vi "EISExample.vi"() -> ()   [LabVIEW 2025]
uses:
  PalmSens/PalmSens.lvclass
  PalmSens/MeasurementResults.ctl
  PalmSens/LiveCurveResult.ctl
  E:/PSCode/PalmSens_SDK/labview/PalmSens/Libraries/PalmSens.Core.Simplified.LabVIEW.dll
  PalmSens/Libraries/PalmSens.Core.Simplified.LabVIEW.dll
panel:
  out "Method Indicator":refnum<k24>
  out "Results":T1
  out "Array":string[](array[string])
  out "Is Measuring":bool
  in  "PalmSens.lvclass":refnum<class "PalmSens.lvclass">
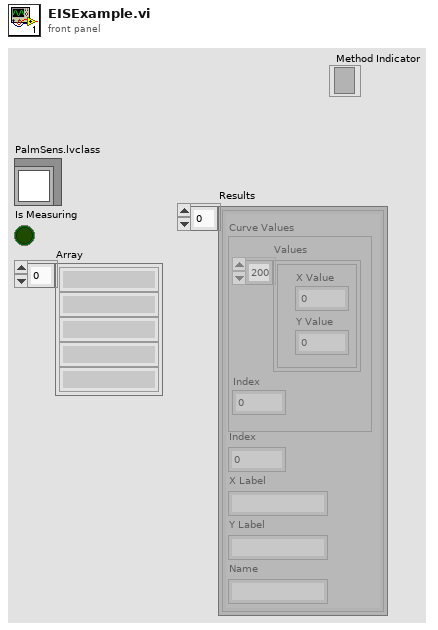
[diagram p1: front panel]
types:
  T1 = typedef "MeasurementResults.ctl" = T2[]
  T2 = typedef "LiveCurveResult.ctl" = cluster{"X Label":string, "Y Label":string, "Name":string, "Index":i16, "Curve Values":cluster{"Values":cluster{"X Value":dbl, "Y Value":dbl}[], "Index":i16}}
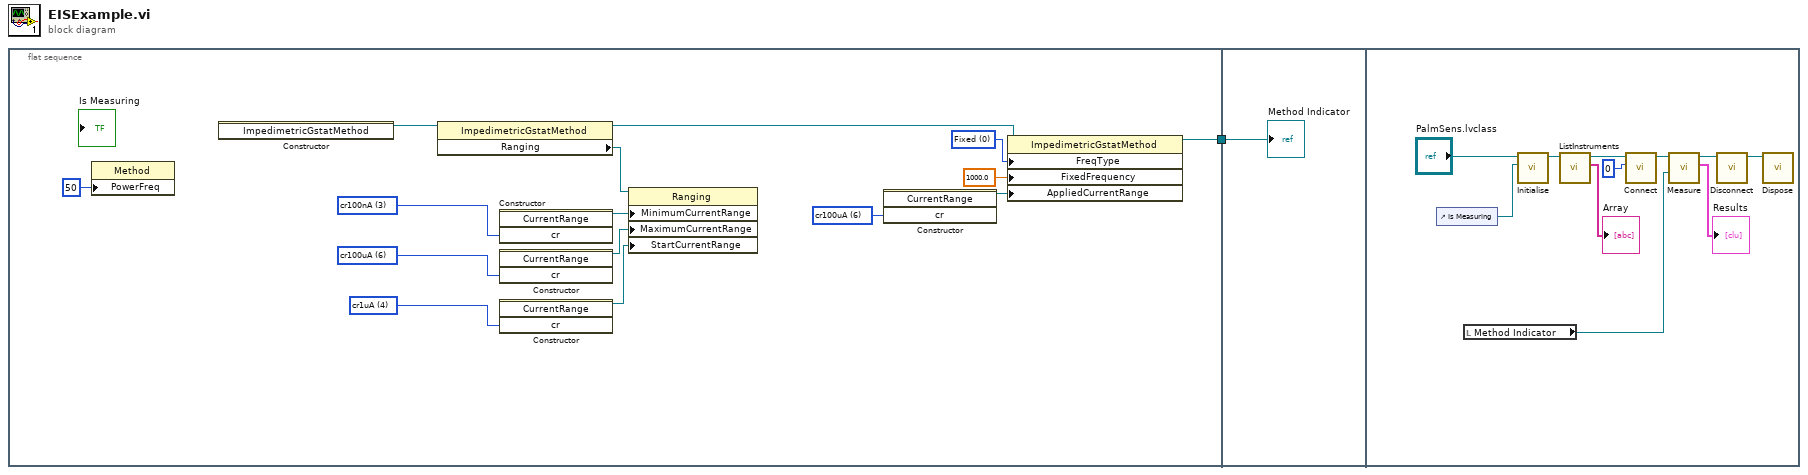
[diagram p0: block diagram]
diagram:
  n1 = flat-sequence {
    tunnel: [w2] -> w1
    tunnel: w1 -> [w17]
    frame #0 {
      w8 = 6 items=["cr100pA"=0, "cr1nA"=1, "cr10nA"=2, "cr100nA"=3, "cr1uA"=4, "cr10uA"=5, "cr100uA"=6, "cr1mA"=7, "cr10mA"=8, "cr100mA"=9, "cr2uA"=10, "cr4uA"=11, "cr8uA"=12, "cr16uA"=13, "cr32uA"=14, "cr125uA"=17, "cr250uA"=18, "cr500uA"=19, "cr5mA"=20, "cr6uA"=21, "cr13uA"=22, "cr25uA"=23, "cr50uA"=24, "cr200uA"=25, "cr63uA"=26, "cr1mA_shunt"=27, "cr10mA_shunt"=28, "cr100mA_shunt"=29, "cr1A"=30, "cr2500uA"=31] ("cr")
      w7 = 0 items=["Fixed", "Scan"] ("FreqType")
      w5 = 4 items=["cr100pA"=0, "cr1nA"=1, "cr10nA"=2, "cr100nA"=3, "cr1uA"=4, "cr10uA"=5, "cr100uA"=6, "cr1mA"=7, "cr10mA"=8, "cr100mA"=9, "cr2uA"=10, "cr4uA"=11, "cr8uA"=12, "cr16uA"=13, "cr32uA"=14, "cr125uA"=17, "cr250uA"=18, "cr500uA"=19, "cr5mA"=20, "cr6uA"=21, "cr13uA"=22, "cr25uA"=23, "cr50uA"=24, "cr200uA"=25, "cr63uA"=26] ("cr")
      w4 = 6 items=["cr100pA"=0, "cr1nA"=1, "cr10nA"=2, "cr100nA"=3, "cr1uA"=4, "cr10uA"=5, "cr100uA"=6, "cr1mA"=7, "cr10mA"=8, "cr100mA"=9, "cr2uA"=10, "cr4uA"=11, "cr8uA"=12, "cr16uA"=13, "cr32uA"=14, "cr125uA"=17, "cr250uA"=18, "cr500uA"=19, "cr5mA"=20, "cr6uA"=21, "cr13uA"=22, "cr25uA"=23, "cr50uA"=24, "cr200uA"=25, "cr63uA"=26] ("cr")
      w3 = 3 items=["cr100pA"=0, "cr1nA"=1, "cr10nA"=2, "cr100nA"=3, "cr1uA"=4, "cr10uA"=5, "cr100uA"=6, "cr1mA"=7, "cr10mA"=8, "cr100mA"=9, "cr2uA"=10, "cr4uA"=11, "cr8uA"=12, "cr16uA"=13, "cr32uA"=14, "cr125uA"=17, "cr250uA"=18, "cr500uA"=19, "cr5mA"=20, "cr6uA"=21, "cr13uA"=22, "cr25uA"=23, "cr50uA"=24, "cr200uA"=25, "cr63uA"=26] ("cr")
      n2 = property class="Method"("PowerFreq"=50) -> ()  [unwired: 2 in, 2 out]
      n3 = constructor class="ImpedimetricGstatMethod"() -> (reference out=w9:refnum<k24>)  [unwired: 3 in, 2 out]
      n4 = property class="ImpedimetricGstatMethod"(reference=w9) -> (reference out=w13:refnum<k24>, "Ranging"=w14:refnum<k24>)  [unwired: 1 in, 1 out]
      n5 = constructor class="CurrentRange"("cr"=w3) -> (reference out=w10:refnum<k24>)  [unwired: 3 in, 3 out]
      n6 = constructor class="CurrentRange"("cr"=w4) -> (reference out=w12:refnum<k24>)  [unwired: 3 in, 3 out]
      n7 = constructor class="CurrentRange"("cr"=w5) -> (reference out=w11:refnum<k24>)  [unwired: 3 in, 3 out]
      n8 = property class="Ranging"(reference=w14, "MinimumCurrentRange"=w10, "MaximumCurrentRange"=w12, "StartCurrentRange"=w11) -> ()  [unwired: 1 in, 2 out]
      n9 = constructor class="CurrentRange"("cr"=w8) -> (reference out=w15:refnum<k24>)  [unwired: 3 in, 3 out]
      n10 = property class="ImpedimetricGstatMethod"(reference=w13, "FreqType"=w7, "FixedFrequency"=sgl 1000.0, "AppliedCurrentRange"=w15) -> (reference out=w2:refnum<k24>)  [unwired: 1 in, 1 out]
    }
    frame #1 {
      "Method Indicator" <- w17
    }
    frame #2 {
      n11 = control-ref of="Is Measuring"() -> (w21:refnum<vi>)
      n12 = local read "Method Indicator"() -> (w18:refnum<k24>)
      n13 = call-dynamic "Initialise.vi"("Is Measuring Refnum"=w21, "PalmSens in"="PalmSens.lvclass") -> ("PalmSens out"=w22:refnum<class "PalmSens.lvclass">)  [unwired: 8 in, 1 out]
      n14 = call-dynamic "ListInstruments.vi"("PalmSens in"=w22) -> ("Array"=→"Array":string[], "PalmSens out"=w24:refnum<class "PalmSens.lvclass">)  [unwired: 8 in, 1 out]
      n15 = call-dynamic "Connect.vi"("Instrument Index"=0, "PalmSens in"=w24) -> ("PalmSens out"=w28:refnum<class "PalmSens.lvclass">)  [unwired: 8 in, 1 out]
      n16 = call-dynamic "Measure.vi"("Method .NET Refnum"=w18, "PalmSens in"=w28) -> ("Curves"=→"Results":T1, "PalmSens out"=w27:refnum<class "PalmSens.lvclass">)  [unwired: 2 in, 2 out]
      n17 = call-dynamic "Disconnect.vi"("PalmSens in"=w27) -> ("PalmSens out"=w25:refnum<class "PalmSens.lvclass">)  [unwired: 9 in, 1 out]
      n18 = call-dynamic "Dispose.vi"("PalmSens in"=w25) -> ()  [unwired: 9 in, 2 out]
    }
  }
